vi "wait to fill the buffer.vi"(8 "error in (no error)":errorcluster, 9 "signal out":waveform(dbl), 11 "task in":refnum<k21>) -> (0 "error out":errorcluster, 3 "task out":refnum<k21>)   [LabVIEW 2014]
uses:
  <resource>/objmgr/daqmx.rc
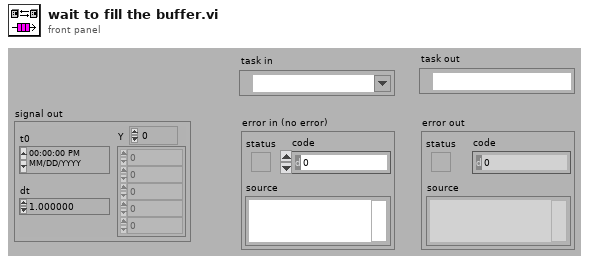
[diagram p1: front panel]
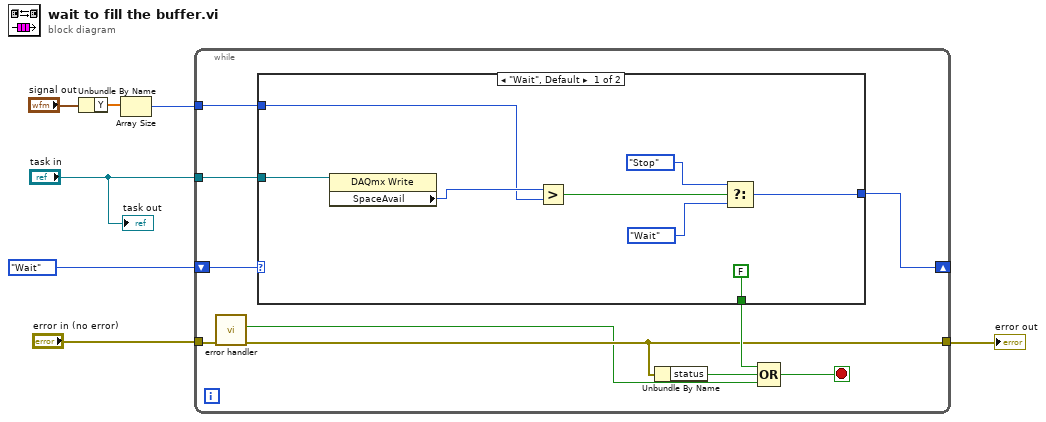
[diagram p0: block diagram]
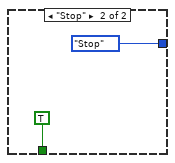
[diagram p2: hidden frame]
diagram:
  n1 = Unbundle By Name("signal out") -> ("Y"=w2:dbl[])
  n2 = Array Size(array=w2) -> (size(s)=w1:i32)
  n3 = while {
    shift-right: [w16] -> _
    shift-left: enum16{"Wait", "Stop"}."Wait" ("Status") -> [w17]
    tunnel: [w9] -> w6
    tunnel: "error in (no error)" -> [w10]
    tunnel: "task in" -> [w12]
    tunnel: w1 -> [w11]
    stop <- w13 stop-if-true
    n4 = call "error handler.vi"("error in (no error)"=w10) -> ("error out"=w9:errorcluster, "error"=w8:bool)  [unwired: 9 in]
    n5 = case shown="\"Wait\", Default" w17 {
      tunnel: [w23 enum16{"Wait", "Stop"}."Stop" ("Status 2")] -> w16
      tunnel: [FALSE TRUE] -> w14
      tunnel: w12 -> [w21 _]
      tunnel: w11 -> [w19 _]
      frame "Wait", Default {
        n6 = property class="DAQmx Write"(reference=w21) -> ("SpaceAvail"=w20:u32)  [unwired: 1 in, 2 out]
        n7 = Greater?(x=w20, y=w19) -> (0:w18:bool)
        n8 = Select(t=enum16{"Wait", "Stop"}."Stop" ("Status 2"), s=w18, f=enum16{"Wait", "Stop"}."Wait" ("Status 2")) -> (s? t:f=w23:enum16{"Wait", "Stop"})
      }
      frame "Stop" {
      }
    }
    n9 = Unbundle By Name(w9) -> ("status"=w15:bool)
    n10 = Compound Arithmetic op=OR(w14, w15, w8) -> (w13:bool)
  }
  "error out" <- w6
  "task out" <- "task in"
